vi "Test_Performance_Gen_Noisy_Img-1.vi"() -> ()   [LabVIEW 2020]
panel:
  in  "Constant\nGeneration":bool
  in  "Generation \nSubprograms":T1(ring)
  out "ms for U16 pixels\nto img transfer":u32
  out "Image":T2(plugin-control)
  in  "stop":bool
  in  "Generate Pic":bool
  out "Raw Pixel Values":u16[][](graph)
  out "ms for generation\nof single noisy img":u32
  in  "Width":i32=2 min=2 max=10000 step=1
  in  "Height":i32=2 min=2 max=5000 step=1
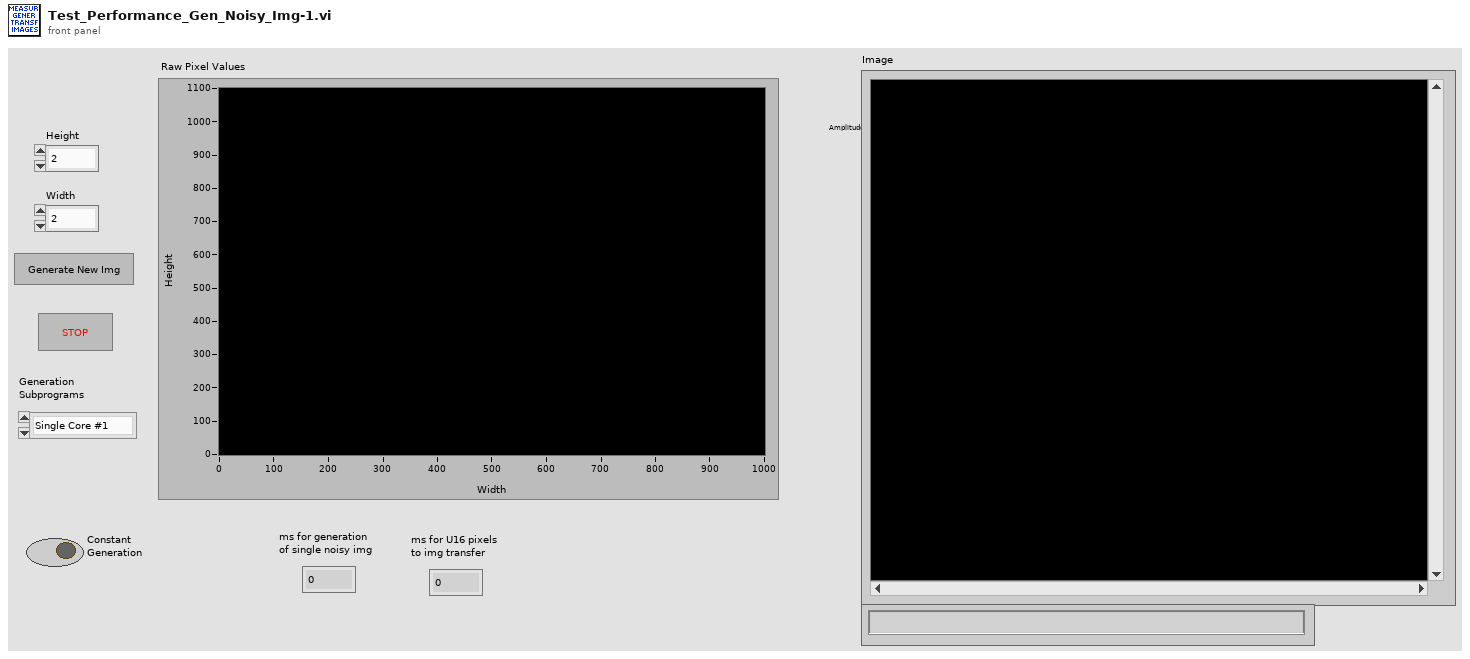
[diagram p1: front panel]
types:
  T1 = enum16{"Single Core #1", "Single Core #2", "Multiple Cores #3"}
  T2 = typedef "IMAQ Image.ctl" = refnum<image>
  T3 = typedef "Image Type" = u32
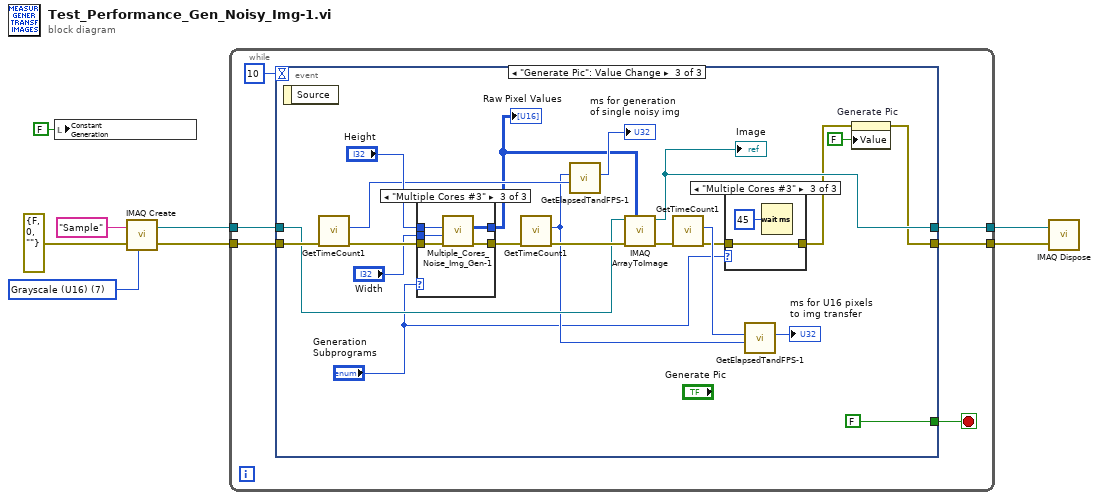
[diagram p0: block diagram]
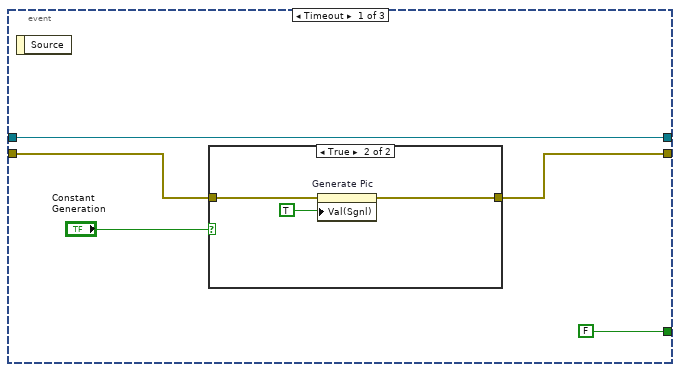
[diagram p2: hidden frame]
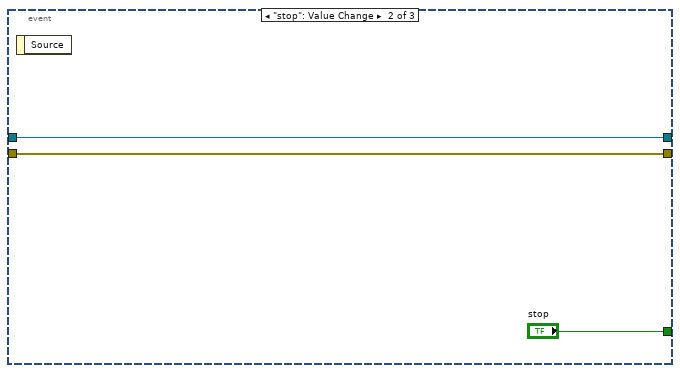
[diagram p4: hidden frame]
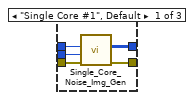
[diagram p7: hidden frame]
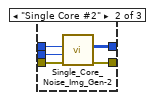
[diagram p8: hidden frame]
diagram:
  w6 = T3 7 items=["Grayscale (U8)", "Grayscale (I16)", "Grayscale (SGL)", "Complex (CSG)", "RGB (U32)", "HSL (U32)", "RGB (U64)", "Grayscale (U16)"] ("Image Type")
  n1 = local write "Constant\nGeneration"(FALSE ("Constant \nGeneration")) -> ()
  n2 = call "IMAQ Create"("Image Name"="Sample", "Image Type"=w6, "error in (no error)"=errorcluster {"status"=FALSE, "code"=0, "source"=""}) -> ("New Image"=w3:T2, "error out"=w5:errorcluster)  [unwired: 2 in]
  n3 = while {
    tunnel: w5 -> [w14]
    tunnel: [w13] -> w4
    tunnel: w3 -> [w12]
    tunnel: [w11] -> w2
    stop <- w10 stop-if-true
    n4 = event shown="[2] \"Generate Pic\": Value Change" {
      selector: _ -> [_ _ _]
      dyn-events: _ -> [_ _ _]
      timeout: 10 -> [_ _ _]
      tunnel: w14 -> [w16 w25 w40]
      tunnel: [w15 w25 w31] -> w13
      tunnel: w12 -> [w19 w24 w38]
      tunnel: [w19 w24 w35] -> w11
      tunnel: [FALSE ("stop") "stop" FALSE ("stop")] -> w10
      event Timeout {
        n5 = event-data() -> ()  [unwired: 1 in, 1 out]
        n6 = case shown="True" "Constant\nGeneration" {
          tunnel: w16 -> [w20 w23]
          tunnel: [w20 w22] -> w15
          frame False {
          }
          frame True {
            n7 = property on="Generate Pic" class="Bool (strict)"(error in=w23, "Val(Sgnl)"=TRUE ("Value (Signaling)")) -> (error out=w22:errorcluster)  [unwired: 1 in, 1 out]
          }
        }
      }
      event "stop": Value Change {
        n8 = event-data() -> ()  [unwired: 1 in, 1 out]
      }
      event "Generate Pic": Value Change {
        n9 = event-data() -> ()  [unwired: 1 in, 1 out]
        n10 = call "GetTimeCount1.vi"("error IN"=w40) -> ("error OUT"=w46:errorcluster, "[OUT] Timer Count"=w43:u32)  [unwired: 9 in]
        n11 = case shown="\"Multiple Cores #3\"" "Generation \nSubprograms" {
          tunnel: w46 -> [w56 w61 w66]
          tunnel: "Height" -> [w55 w59 w63]
          tunnel: [w54 w58 w65] -> w44
          tunnel: "Width" -> [w53 w60 w62]
          tunnel: [w52 w57 w64] -> w37
          frame "Single Core #1", Default {
            n12 = call "Single_Core_Noise_Img_Gen.vi"("error IN"=w56, "[IN] Width"=w53, "[IN] Height"=w55) -> ("error OUT"=w54:errorcluster, "[OUT] U16 Pixel Img"=w52:u16[][])  [unwired: 7 in]
          }
          frame "Single Core #2" {
            n13 = call "Single_Core_Noise_Img_Gen-2.vi"("error IN"=w61, "[IN] Width"=w60, "[IN] Height"=w59) -> ("error OUT"=w58:errorcluster, "[OUT] U16 Pixel Img"=w57:u16[][])  [unwired: 7 in]
          }
          frame "Multiple Cores #3" {
            n14 = call "Multiple_Cores_Noise_Img_Gen-1.vi"("error IN"=w66, "[IN] Width"=w62, "[IN] Height"=w63) -> ("error OUT"=w65:errorcluster, "[OUT] U16 Pixel Img"=w64:u16[][])  [unwired: 7 in]
          }
        }
        "Raw Pixel Values" <- w37
        n15 = call "GetTimeCount1.vi"("error IN"=w44) -> ("error OUT"=w39:errorcluster, "[OUT] Timer Count"=w33:u32)  [unwired: 9 in]
        n16 = call "GetElapsedTandFPS-1.vi"("[IN] Timer Count Before ALL [ms]"=w43, "[IN] Timer Count After ALL [ms]"=w33) -> ("[OUT] Elapsed time [ms]"=→"ms for generation\nof single noisy img":u32)  [unwired: 3 in, 2 out]
        n17 = call "IMAQ ArrayToImage"("Image Pixels (U16)"=w37, "error in (no error)"=w39, "Image"=w38) -> ("error out"=w36:errorcluster, "Image Out"=w35:T2)  [unwired: 7 in]
        "Image" <- w35
        n18 = call "GetTimeCount1.vi"("error IN"=w36) -> ("error OUT"=w28:errorcluster, "[OUT] Timer Count"=w34:u32)  [unwired: 9 in]
        n19 = case shown="\"Multiple Cores #3\"" "Generation \nSubprograms" {
          tunnel: w28 -> [w48 w49 w50]
          tunnel: [w48 w49 w50] -> w27
          frame "Single Core #1", Default {
          }
          frame "Single Core #2" {
          }
          frame "Multiple Cores #3" {
            n20 = Wait (ms)(milliseconds to wait=u32 45) -> ()  [unwired: 1 out]
          }
        }
        n21 = call "GetElapsedTandFPS-1.vi"("[IN] Timer Count Before ALL [ms]"=w33, "[IN] Timer Count After ALL [ms]"=w34) -> ("[OUT] Elapsed time [ms]"=→"ms for U16 pixels\nto img transfer":u32)  [unwired: 3 in, 2 out]
        n22 = property on="Generate Pic" class="Bool (strict)"(error in=w27, "Value"=FALSE ("Generate Pic")) -> (error out=w31:errorcluster)  [unwired: 1 in, 1 out]
      }
    }
  }
  n23 = call "IMAQ Dispose"("Image"=w2, "error in (no error)"=w4) -> ()  [unwired: 4 in, 1 out]
